vi "Mech Calculate_Drive_Power_Nemo_Style.vi"(7 "Reverse":bool, 8 "Deadband (10)":i8=10 min=0 max=100 step=1, 10 "Controller State":T1={"Left X"=0, "Left Y"=0, "Right X"=0, "Right Y"=0, "Button Encoding 9-12"=0, "Button Encoding 1-8"=0, "POV"=-1} {"POV" items=["None"=-1, "POV Up"=0, "POV Up Right"=1, "POV Right"=2, "POV Down Right"=3, "POV Down"=4, "POV Down Left"=5, "POV Left"=6, "POV Up Left"=7]}, 11 "Power Level (100)":i8=100 min=-100 max=100) -> (0 "Right Rear Power":i8, 1 "Right Front Power":i8, 2 "Left Rear Power":i8, 3 "Left Front Power":i8)   [LabVIEW 2012]
doc: "Determines the amount of power to apply to a set of motors according to the x and y values of two joysticks on a game controller for a mecanum drive train.\n\n<B>Inputs</B>\n<B>Power Level</B> specifies the maximum amount of power to apply to the motor. For example, a value of 50 scales the fuznge of the joystick to a range of -50 to 50. A negative value drives the motor with the same power as its equivalent positive number but in the opposite direction. You can specify a value between -100 and 100. A value of 0 specifies the motor does not move. The default is 50.\n<B>Controller State</B> specifies the values of the joystick axes and button states of the game controller.\n<B>Deadband</B> specifies the joystick values that the VI treats as zero. When the position of the joystick is within the range you specify, the VI considers the joystick to be at position 0. The default range is -10 to 10.\n\n<B>Outputs</B>\n<B>Left Front Motor Power</B> returns the amount of power to apply to the left front motor. \n<B>Left Rear Motor Power</B> returns the amount of power to apply to the left rear motor. \n<B>Right Front Motor Power</B> returns the amount of power to apply to the right front motor.\n<B>Right Rear Motor Power</B> returns the amount of power to apply to the right rear motor.\n\nLF power = Ly + Rx + Lx\nRF power = Ly - Rx - Lx\nLR power = Ly + Rx - Lx\nRR power = Ly - Rx +Lx"
uses:
  <vilib>/FTC/FTC ControllerState.ctl
  <vilib>/FTC/FTC POVState.ctl
  <vilib>/NXT/Dual Mode Library/prims/inRangeAndCoerce/inRangeAndCoerce_float.vi
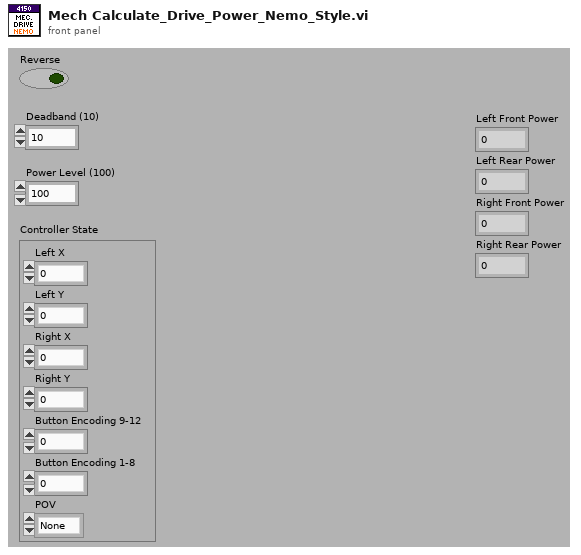
[diagram p1: front panel]
types:
  T1 = typedef "FTC ControllerState.ctl" = cluster{"Left X":i8, "Left Y":i8, "Right X":i8, "Right Y":i8, "Button Encoding 9-12":u8, "Button Encoding 1-8":u8, "POV":T2}
  T2 = typedef "FTC POVState.ctl" = i8
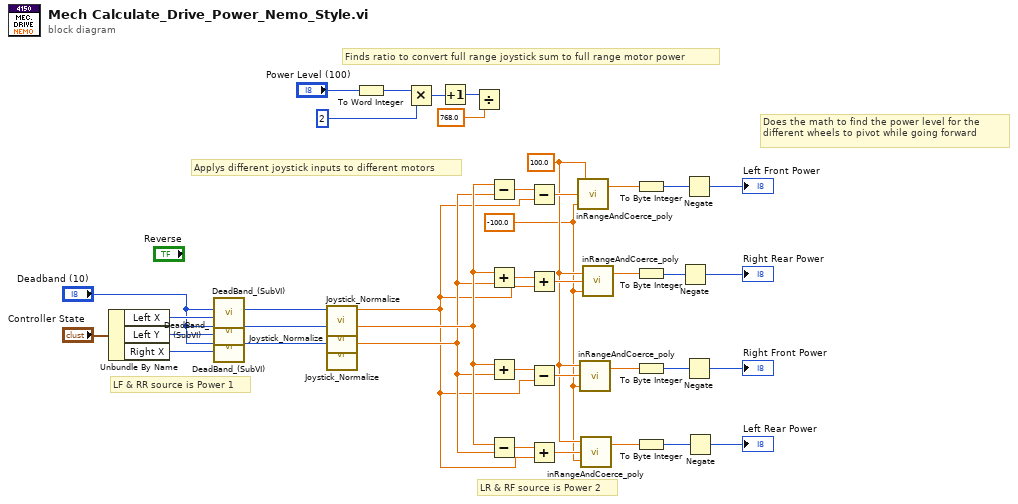
[diagram p0: block diagram]
diagram:
  w15 = sgl -100.0 ("lower limit")
  w16 = sgl 100.0 ("upper limit")
  # "Does the math to find the power level for the \ndifferent wheels to pivot while going forward"
  # "Applys different joystick inputs to different motors"
  # "Finds ratio to convert full range joystick sum to full range motor power"
  # "LR & RF source is Power 2"
  # "LF & RR source is Power 1"
  n1 = Unbundle By Name("Controller State") -> ("Left X"=w38:i8, "Left Y"=w36:i8, "Right X"=w35:i8)
  n2 = call "DeadBand_(SubVI).vi"("Axis In"=w38, "Deadband (10)"="Deadband (10)") -> ("Axis out"=w1:i8)  [unwired: 9 in]
  n3 = call "DeadBand_(SubVI).vi"("Axis In"=w36, "Deadband (10)"="Deadband (10)") -> ("Axis out"=w9:i8)  [unwired: 9 in]
  n4 = call "DeadBand_(SubVI).vi"("Axis In"=w35, "Deadband (10)"="Deadband (10)") -> ("Axis out"=w7:i8)  [unwired: 9 in]
  n5 = call "Joystick_Normalize.vi"("Joystick In"=w1) -> ("Norm Out"=w6:dbl)  [unwired: 10 in]
  n6 = call "Joystick_Normalize.vi"("Joystick In"=w9) -> ("Norm Out"=w10:dbl)  [unwired: 10 in]
  n7 = call "Joystick_Normalize.vi"("Joystick In"=w7) -> ("Norm Out"=w8:dbl)  [unwired: 10 in]
  n8 = To Word Integer(number="Power Level (100)") -> (16bit integer=w21:i16)
  n9 = Multiply(x=w21, y=i16 2) -> (x*y=w24:i16)
  n10 = Increment(x=w24) -> (x+1=w23:i16)
  n11 = Divide(x=w23, y=768.0) -> ()  [unwired: 1 out]
  n12 = Subtract(x=w10, y=w8) -> (x-y=w34:dbl)
  n13 = Add(x=w10, y=w8) -> (x+y=w33:dbl)
  n14 = Add(x=w10, y=w8) -> (x+y=w32:dbl)
  n15 = Subtract(x=w10, y=w8) -> (x-y=w31:dbl)
  n16 = Subtract(x=w34, y=w6) -> (x-y=w20:dbl)
  n17 = Add(x=w33, y=w6) -> (x+y=w17:dbl)
  n18 = Subtract(x=w32, y=w6) -> (x-y=w18:dbl)
  n19 = Add(x=w31, y=w6) -> (x+y=w19:dbl)
  n20 = call-poly <vilib>:"inRangeAndCoerce_poly.vi"("lower limit"=w15, "x"=w20, "upper limit"=w16) -> ("coerced(x)"=w11:sgl)  [unwired: 1 out]
  n21 = call-poly <vilib>:"inRangeAndCoerce_poly.vi"("lower limit"=w15, "x"=w18, "upper limit"=w16) -> ("coerced(x)"=w13:sgl)  [unwired: 1 out]
  n22 = call-poly <vilib>:"inRangeAndCoerce_poly.vi"("lower limit"=w15, "x"=w19, "upper limit"=w16) -> ("coerced(x)"=w12:sgl)  [unwired: 1 out]
  n23 = call-poly <vilib>:"inRangeAndCoerce_poly.vi"("lower limit"=w15, "x"=w17, "upper limit"=w16) -> ("coerced(x)"=w14:sgl)  [unwired: 1 out]
  n24 = To Byte Integer(number=w11) -> (8bit integer=w30:i8)
  n25 = To Byte Integer(number=w14) -> (8bit integer=w29:i8)
  n26 = To Byte Integer(number=w13) -> (8bit integer=w28:i8)
  n27 = To Byte Integer(number=w12) -> (8bit integer=w27:i8)
  n28 = Negate(x=w29) -> (-x=→"Right Rear Power":i8)
  n29 = Negate(x=w30) -> (-x=→"Left Front Power":i8)
  n30 = Negate(x=w28) -> (-x=→"Right Front Power":i8)
  n31 = Negate(x=w27) -> (-x=→"Left Rear Power":i8)
